vi "Gripper call.vi"(10 "Buttons Pressed":bool[](array[boolean])) -> ()   [LabVIEW 2017]
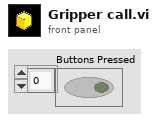
[diagram p1: front panel]
types:
  T1 = typedef "Command Status Info.ctl" = cluster{"Name":string, "Status":T2, "notifier out":T3}
  T2 = typedef "Completion Status.ctl" = enum16{"Successful", "Aborted", "Incomplete"}
  T3 = typedef "Completion Notifier.ctl" = refnum<notifier>
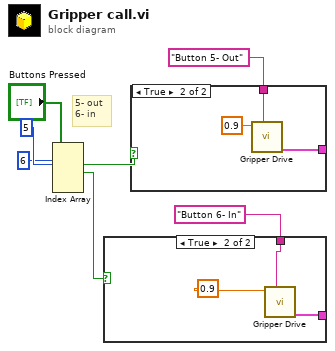
[diagram p0: block diagram]
diagram:
  # "5- out \n6- in"
  n1 = Index Array(array="Buttons Pressed", index #1=5 ("index"), index #2=6 ("index")) -> (element #1=w7:bool, element #2=w6:bool)  [unwired: 2 in, 2 out]
  n2 = case shown="True" w6 {
    tunnel: "Button 6- In" ("Description") -> [_ w9]
    tunnel: [_ w8] -> _
    frame False {
    }
    frame True {
      n3 = call "Gripper Drive.vi"("Description"=w9, "Right Motor"=0.9 ("Setpoint")) -> ("Command Info Out"=w8:T1)  [unwired: 9 in]
    }
  }
  n4 = case shown="True" w7 {
    tunnel: [_ w12] -> _
    tunnel: "Button 5- Out" ("Description") -> [_ w11]
    frame False {
    }
    frame True {
      n5 = call "Gripper Drive.vi"("Description"=w11, "Right Motor"=0.9 ("Setpoint")) -> ("Command Info Out"=w12:T1)  [unwired: 9 in]
    }
  }
